vi "initDAQ.vi"(8 "clock source":i32(ring) items=["OnboardClock", "ExternalClock", "NoClock"], 9 "Maximum Value":dbl=10.0 format="%0.2f", 10 "Minimum Value":dbl format="%0.2f", 11 "Physical Channel":refnum<k21>="Dev0/Ai0:1") -> ()   [LabVIEW 2011]
uses:
  <vilib>/ULx/Create Channel.llb/ULx Create Channel (AI-Voltage-Basic).vi
  <vilib>/ULx/Create Channel.llb/ULx Create Channel (DO-Digital Output).vi
  <vilib>/ULx/Write.llb/ULx Write (Digital 1D Bool 1Chan 1Samp).vi
  <vilib>/ULx/Timing.llb/ULx Timing (Sample Clock).vi
  GlobalDAQ.vi
panel:
  in  "valve data":bool[](array[boolean])=[FALSE, FALSE, FALSE, FALSE, FALSE, FALSE, FALSE, FALSE]
  in  "output lines":refnum<k21>="Dev0/1stPortA/Do0:7"
  out "sampling rate":dbl=400.0
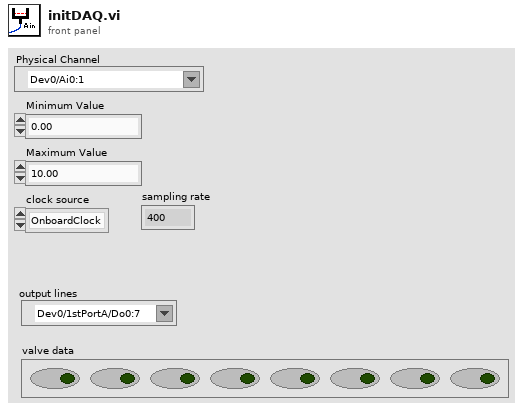
[diagram p1: front panel]
types:
  T1 = typedef "Semaphore RefNum" = refnum<k1>
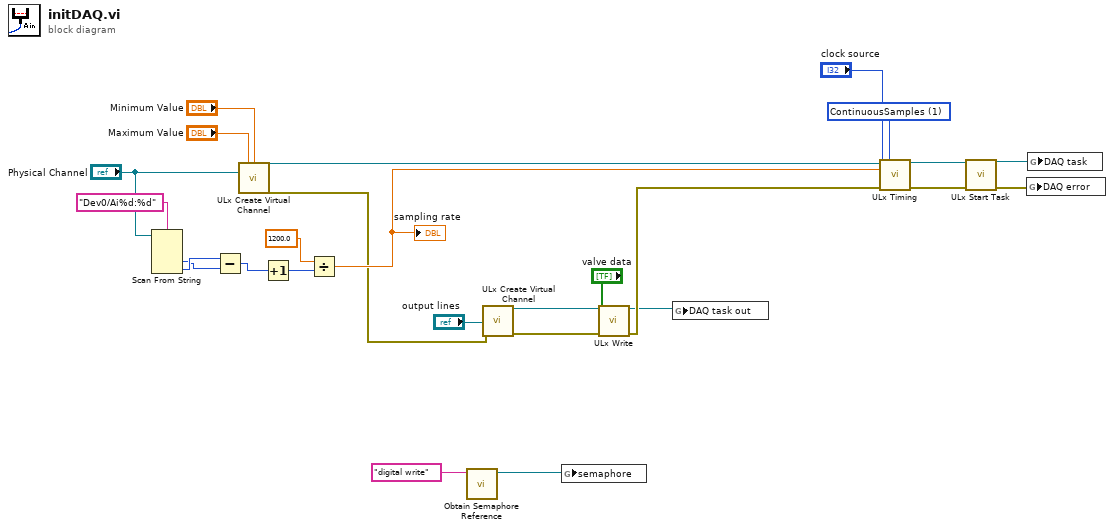
[diagram p0: block diagram]
diagram:
  w23 = 1 items=["FiniteSamples", "ContinuousSamples"] ("sample mode")
  n1 = Scan From String(format string="Dev0/Ai%d:%d", input string="Physical Channel") -> (output 1=w16:i32, output 2=w17:i32)  [unwired: 4 in, 3 out]
  n2 = Subtract(x=w17, y=w16) -> (x-y=w13:i32)
  n3 = call-poly <vilib>:"ULx Create Virtual Channel.vi"("maximum value"="Maximum Value", "minimum value"="Minimum Value", "physical channels"="Physical Channel") -> ("task out"=w26:refnum<k24>, "error out"=w10:errorcluster)  [unwired: 11 in]
  n4 = Increment(x=w13) -> (x+1=w12:i32)
  n5 = Divide(x=1200.0, y=w12) -> (x/y=w14:dbl)
  "sampling rate" <- w14
  n6 = call <vilib>:"Obtain Semaphore Reference.vi"("name (unnamed)"="digital write") -> ("semaphore"=w1:T1)  [unwired: 4 in, 2 out]
  n7 = call-poly <vilib>:"ULx Create Virtual Channel.vi"("lines"="output lines", "error in"=w10) -> ("task out"=w9:refnum<k24>, "error out"=w8:errorcluster)  [unwired: 12 in]
  n8 = global write "GlobalDAQ.vi" "semaphore"(w1) -> ()
  n9 = call-poly <vilib>:"ULx Write.vi"("task in"=w9, "data"="valve data", "error in"=w8) -> ("task out"=w6:refnum<k24>, "error out"=w7:errorcluster)  [unwired: 10 in, 1 out]
  n10 = global write "GlobalDAQ.vi" "DAQ task out"(w6) -> ()
  n11 = call-poly <vilib>:"ULx Timing.vi"("task in"=w26, "sample mode"=w23, "rate"=w14, "clock source"="clock source", "error in"=w7) -> ("task out"=w25:refnum<k24>, "error out"=w24:errorcluster)  [unwired: 9 in]
  n12 = call <vilib>:"ULx Start Task.vi"("task in"=w25, "error in"=w24) -> ("task out"=w4:refnum<k24>, "error out"=w3:errorcluster)  [unwired: 12 in]
  n13 = global write "GlobalDAQ.vi" "DAQ error"(w3) -> ()
  n14 = global write "GlobalDAQ.vi" "DAQ task"(w4) -> ()
